vi "Read Current VFD.vi"(8 "error In":errorcluster) -> (0 "error out":errorcluster, 3 "Current":dbl format="%#_13g")   [LabVIEW 2026, in "VFD Library.lvlib"]
uses:
  VFD Library.lvlib
  Private/State Selection FGV.ctl
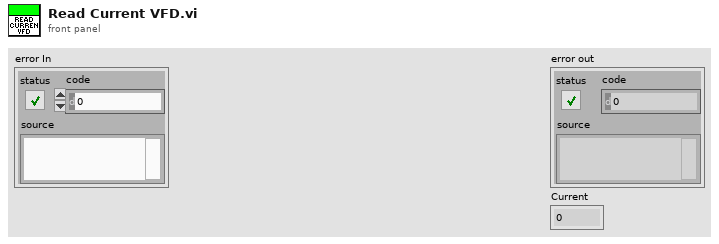
[diagram p1: front panel]
types:
  T1 = typedef "State Selection FGV.ctl" = enum16{"Initilize", "Write Reg", "Write Multiple Reg", "Read Reg", "Write Coil", "Read Coil", "Reset", "Close"}
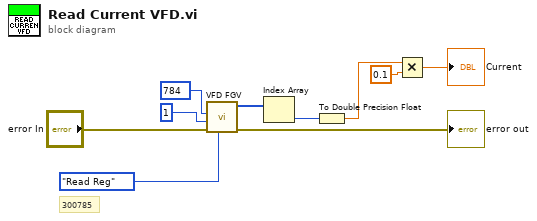
[diagram p0: block diagram]
diagram:
  # "300785"
  n1 = call "VFD FGV.vi"("State"=State_Selection_FGV."Read Reg", "error In"="error In", "value"=u16 1, "address"=u16 784) -> ("error out"=→"error out":errorcluster, "Registers"=w2:u16[])  [unwired: 5 in, 1 out]
  n2 = Index Array(array=w2) -> (element=w5:u16)  [unwired: 1 in]
  n3 = To Double Precision Float(number=w5) -> (double precision float=w1:dbl)
  n4 = Multiply(x=w1, y=0.1) -> (x*y=→"Current":dbl)
